vi "Unmodified_LuaL_Buffer.vi"(11 "Modified_LuaL_Buffer 2":T1) -> (3 "LuaL_Buffer *B":T2)   [LabVIEW 2011]
types:
  T1 = cluster{"U*8 Array":cluster{"U*8 Array[0]":u8}, "size_t size":u32, "size_t n":u32, "lua_State *L":u64, "U*8 Array":cluster{"U*8 Array[0]":u8, "U*8 Array[1]":u8, "U*8 Array[2]":u8, "U*8 Array[3]":u8, "U*8 Array[4]":u8, "U*8 Array[5]":u8, "U*8 Array[6]":u8, "U*8 Array[7]":u8, "U*8 Array[8]":u8, "U*8 Array[9]":u8}}
  T2 = cluster{"char *b":string, "size_t size":u32, "size_t n":u32, "lua_State *L":u64, "char initb[LUAL_BUFFERSIZE]":string}
  T3 = cluster{"U*8 Array[0]":u8, "U*8 Array[1]":u8, "U*8 Array[2]":u8, "U*8 Array[3]":u8, "U*8 Array[4]":u8, "U*8 Array[5]":u8, "U*8 Array[6]":u8, "U*8 Array[7]":u8, "U*8 Array[8]":u8, "U*8 Array[9]":u8}
  T4 = cluster{string, "size_t size":u32, "size_t n":u32, "lua_State *L":u64, string}
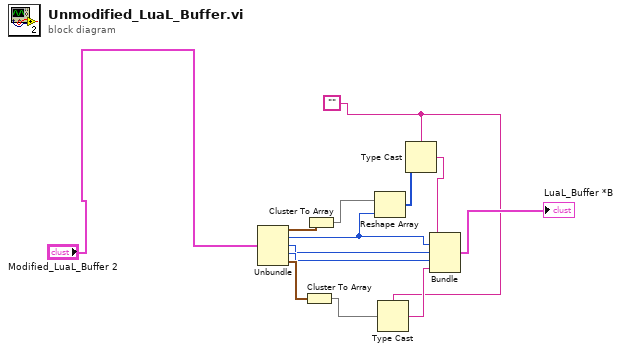
[diagram p0: block diagram]
diagram:
  w11 = ""
  n1 = Unbundle("Modified_LuaL_Buffer 2") -> ("U*8 Array"=w2:cluster{"U*8 Array[0]":u8}, "size_t size"=w4:u32, "size_t n"=w5:u32, "lua_State *L"=w6:u64, "U*8 Array"=w9:T3)
  n2 = Cluster To Array(cluster=w9) -> (array=w10:u8[])
  n3 = Cluster To Array(cluster=w2) -> (array=w3:u8[])
  n4 = Reshape Array(w3, w4) -> (w7:u8[])
  n5 = Type Cast(type=w11, x=w10) -> (*(type *) &x=w12:string)
  n6 = Type Cast(type=w11, x=w7) -> (*(type *) &x=w8:string)
  n7 = Bundle(w8, "size_t size"=w4, "size_t n"=w5, "lua_State *L"=w6, w12) -> (→"LuaL_Buffer *B":T4)  [unwired: 1 in]
